vi "open.vi"(8 "error in (no error)":errorcluster caption="错误输入（无错误）", 11 "DAM0200-Relay 输入":refnum<class "DAM0200-Relay.lvclass">) -> (0 "error out":errorcluster caption="错误输出", 3 "DAM0200-Relay 输出":refnum<class "DAM0200-Relay.lvclass">)   [LabVIEW 2016, in "DAM0200-Relay.lvlib" / "DAM0200-Relay.lvclass"]
uses:
  DAM0200-Relay.lvclass
  DAM0200-Relay.lvclass/DAM0200-Relay.ctl
  <vilib>/Plasmionique/MB Master/MB_Master_Serial/MB_Master_Serial.lvclass
  C:/Program Files (x86)/National Instruments/LabVIEW 2016/vi.lib/Plasmionique/MB Master/MB_Master/MB_Master.lvclass
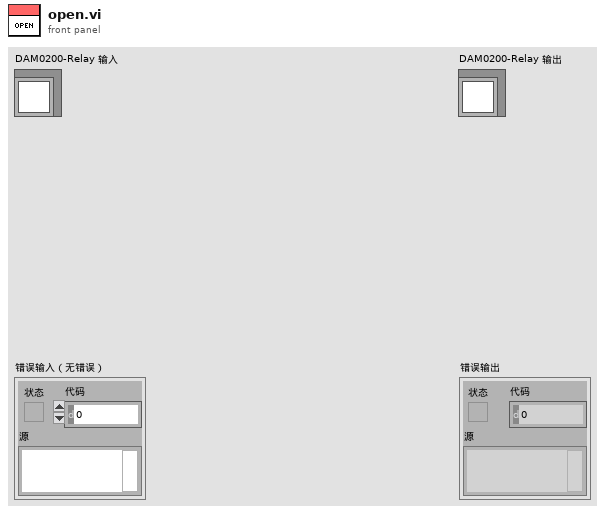
[diagram p1: front panel]
types:
  T1 = cluster{"baud rate (bps)":u32, "stop bits":u16, "parity":u16, "flow control":u16, "timeout":u32, "retries":i32}
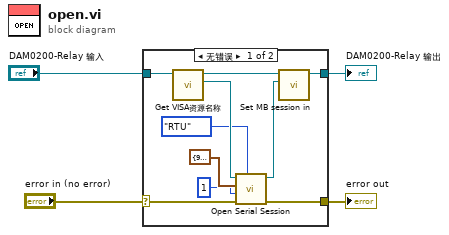
[diagram p0: block diagram]
diagram:
  n1 = case shown="无错误" "error in (no error)" {
    selector: "error in (no error)" -> [w9 w16]
    tunnel: [w8 w16] -> w3
    tunnel: [w5 w15] -> w1
    tunnel: "DAM0200-Relay 输入" -> [w14 w15]
    frame No Error {
      n2 = call "Get VISA资源名称.vi"("DAM0200-Relay in"=w14) -> ("VISA资源名称"=w13:refnum<visa-resource-name>, "DAM0200-Relay out"=w7:refnum<class "DAM0200-Relay.lvclass">)  [unwired: 9 in]
      n3 = call <vilib>:"Open Serial Session.vi"("Mode (RTU)"=enum16{"RTU", "ASCII"}."RTU", "Error in"=w9, "Slave ID"=u8 1, "Serial Config"=T1 {"baud rate (bps)"=9600, "stop bits"=10, "parity"=0, "flow control"=0, "timeout"=1000, "retries"=1}, "VISA Resource"=w13) -> ("Error out"=w8:errorcluster, "MB_Serial session"=w6:refnum<class "MB_Master_Serial.lvclass">)  [unwired: 5 in]
      n4 = call "Set MB session in.vi"("MB Serial Master:MB_Master"=w6, "DAM0200-Relay in"=w7) -> ("DAM0200-Relay out"=w5:refnum<class "DAM0200-Relay.lvclass">)  [unwired: 9 in]
    }
    frame Error {
    }
  }
  "error out" <- w3
  "DAM0200-Relay 输出" <- w1
